vi "DC_Overvoltage_v3.vi"(4 "Polarity":enum16{"Positive", "Negative"}(ring), 5 "Write Task":string="BONTS-93-DC_Link_Input", 6 "# of Channels In":enum16{"1", "2"}(ring), 7 "Read Task":string="BONTS-93-Faults", 8 "error in":errorcluster, 10 "Fault High Threshold":dbl=3.0, 11 "Fault Low Threshold":dbl=0.2) -> (0 "error out":errorcluster, 3 "TS Results":dbl[](array[numeric]))   [LabVIEW 2021]
uses:
  <vilib>/DAQmx/write.llb/DAQmx Write (Analog 1D DBL NChan 1Samp).vi
  <vilib>/DAQmx/read.llb/DAQmx Read (Analog 1D DBL NChan 1Samp).vi
  <vilib>/DAQmx/miscellaneous.llb/DAQmx Fill In Error Info.vi
panel:
  out "Hysteresis":dbl
  out "Fault Out":dbl[](array[numeric]) format="%0.2f"
  in  "Starting Voltage":dbl=4.0
  out "VDC Fault OFF":dbl[](array[numeric])
  in  "Max Voltage":dbl=5.2
  out "VDC Fault ON":dbl[](array[numeric])
  in  "Increments":i32=1000
  # "OV Fault"
  # "Hysteresis"
  # "Fault A"
  # "Fault B"
  # "Fault C"
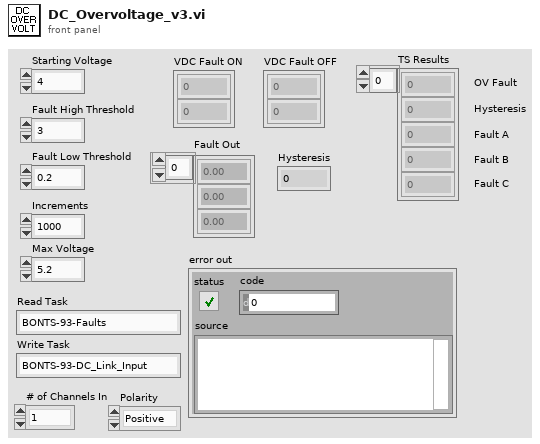
[diagram p1: front panel]
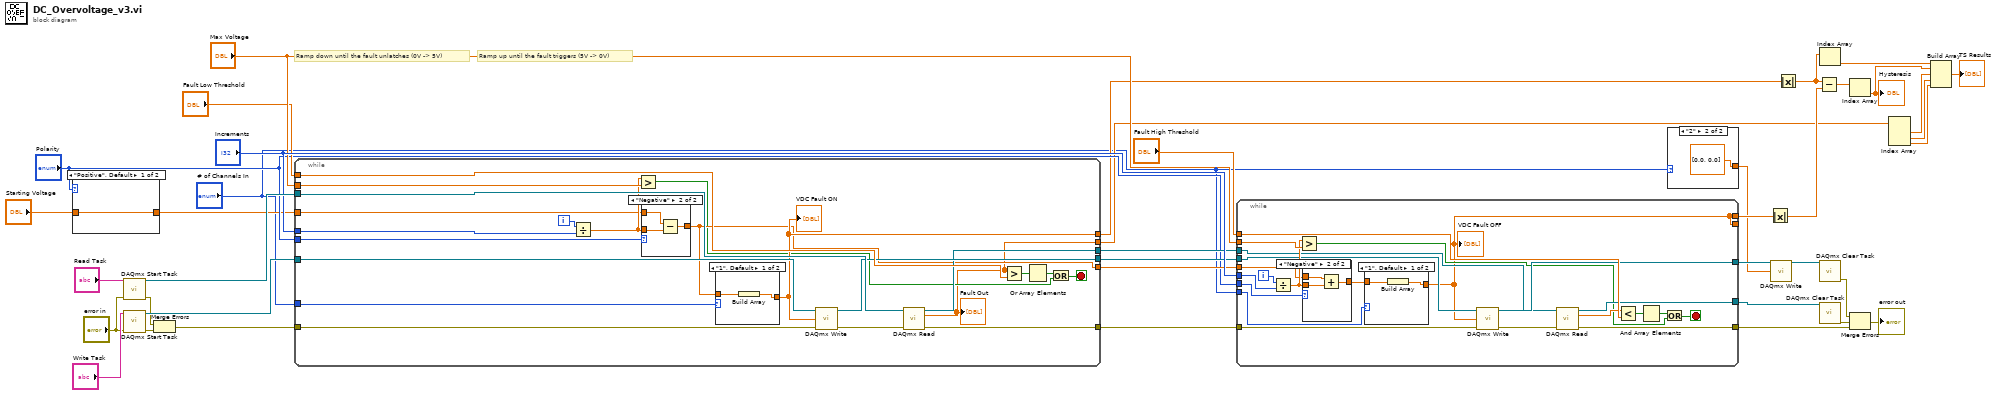
[diagram p0: block diagram]
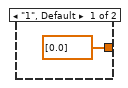
[diagram p2: hidden frame]
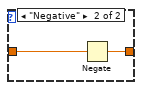
[diagram p3: hidden frame]
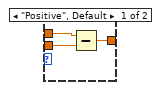
[diagram p4: hidden frame]
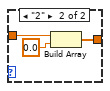
[diagram p5: hidden frame]
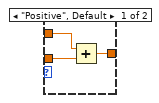
[diagram p6: hidden frame]
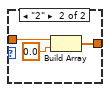
[diagram p7: hidden frame]
diagram:
  # "Ramp down until the fault unlatches (0V -> 5V)"
  # "Ramp up until the fault triggers (5V -> 0V)"
  n1 = case shown="\"Positive\", Default" "Polarity" {
    tunnel: "Starting Voltage" -> [w41 w43]
    tunnel: [w41 w42] -> w15
    frame "Positive", Default {
    }
    frame "Negative" {
      n2 = Negate(x=w43) -> (-x=w42:dbl)
    }
  }
  n3 = call <vilib>:"DAQmx Start Task.vi"("task/channels in"="Read Task", "error in"="error in") -> ("task out"=w37:refnum<k21>, "error out"=w28:errorcluster)  [unwired: 12 in]
  n4 = call <vilib>:"DAQmx Start Task.vi"("task/channels in"="Write Task", "error in"="error in") -> ("task out"=w39:refnum<k21>, "error out"=w27:errorcluster)  [unwired: 12 in]
  n5 = Merge Errors(w28, w27) -> (w29:errorcluster)
  n6 = while {
    tunnel: w37 -> [w65]
    tunnel: w39 -> [w64]
    tunnel: w29 -> [w63]
    tunnel: [w62] -> w25
    tunnel: "Fault Low Threshold" -> [w60]
    tunnel: "Increments" -> [w58]
    tunnel: "Max Voltage" -> [w57]
    tunnel: [w56] -> w24
    tunnel: [w55] -> w23
    tunnel: [w52] -> w22
    tunnel: [w54] -> w13
    tunnel: w15 -> [w51]
    tunnel: "# of Channels In" -> [w50]
    tunnel: "Polarity" -> [w49]
    tunnel: [w44] -> w10
    i -> [w59]
    stop <- w45 stop-if-true
    n7 = Divide(x=w59, y=w58) -> (x/y=w53:dbl)
    n8 = Greater?(x=w53, y=w57) -> (0:w46:bool)
    n9 = case shown="\"Negative\"" w49 {
      tunnel: w53 -> [w67 w71]
      tunnel: [w66 w70] -> w52
      tunnel: w51 -> [w68 w69]
      frame "Positive", Default {
        n10 = Add(x=w68, y=w67) -> (x+y=w66:dbl)
      }
      frame "Negative" {
        n11 = Subtract(x=w69, y=w71) -> (x-y=w70:dbl)
      }
    }
    n12 = case shown="\"1\", Default" w50 {
      tunnel: [w73 w75] -> w54
      tunnel: w52 -> [w72 w74]
      frame "1", Default {
        n13 = Build Array(w72) -> (w73:dbl[])
      }
      frame "2" {
        n14 = Build Array(w74, 0.0 ("element")) -> (w75:dbl[])
      }
    }
    "VDC Fault ON" <- w54
    n15 = call-poly <vilib>:"DAQmx Write.vi"("task/channels in"=w64, "data"=w54, "error in"=w63) -> ("task out"=w56:refnum<k21>, "error out"=w61:errorcluster)  [unwired: 10 in, 1 out]
    n16 = call-poly <vilib>:"DAQmx Read.vi"("task/channels in"=w65, "error in"=w61) -> ("task out"=w55:refnum<k21>, "data"=w44:dbl[], "error out"=w62:errorcluster)  [unwired: 11 in]
    "Fault Out" <- w44
    n17 = Greater?(x=w44, y=w60) -> (0:w48:bool[])
    n18 = Or Array Elements(Boolean array=w48) -> (logical OR=w47:bool)
    n19 = Or(x=w47, y=w46) -> (x .or. y?=w45:bool)
  }
  n20 = while {
    tunnel: [w98] -> w31
    tunnel: "Fault High Threshold" -> [w96]
    tunnel: "Increments" -> [w94]
    tunnel: "Max Voltage" -> [w93]
    tunnel: [w92] -> w34
    tunnel: [w91] -> w21
    tunnel: w25 -> [w90]
    tunnel: w22 -> [w87]
    tunnel: w24 -> [w86]
    tunnel: w23 -> [w85]
    tunnel: [w77] -> _
    tunnel: "# of Channels In" -> [w83]
    tunnel: "Polarity" -> [w82]
    tunnel: [w77] -> w12
    i -> [w95]
    stop <- w78 stop-if-true
    n21 = Divide(x=w95, y=w94) -> (x/y=w88:dbl)
    n22 = Greater?(x=w88, y=w93) -> (0:w79:bool)
    n23 = case shown="\"Negative\"" w82 {
      tunnel: [w101 w102] -> w89
      tunnel: w88 -> [w99 w103]
      tunnel: w87 -> [w100 w104]
      frame "Positive", Default {
        n24 = Subtract(x=w100, y=w99) -> (x-y=w101:dbl)
      }
      frame "Negative" {
        n25 = Add(x=w104, y=w103) -> (x+y=w102:dbl)
      }
    }
    n26 = case shown="\"1\", Default" w83 {
      tunnel: w89 -> [w105 w108]
      tunnel: [w106 w107] -> w77
      frame "1", Default {
        n27 = Build Array(w105) -> (w106:dbl[])
      }
      frame "2" {
        n28 = Build Array(w108, 0.0 ("element")) -> (w107:dbl[])
      }
    }
    "VDC Fault OFF" <- w77
    n29 = call-poly <vilib>:"DAQmx Write.vi"("task/channels in"=w86, "data"=w77, "error in"=w90) -> ("task out"=w91:refnum<k21>, "error out"=w97:errorcluster)  [unwired: 10 in, 1 out]
    n30 = call-poly <vilib>:"DAQmx Read.vi"("task/channels in"=w85, "error in"=w97) -> ("task out"=w92:refnum<k21>, "data"=w84:dbl[], "error out"=w98:errorcluster)  [unwired: 11 in]
    n31 = Less?(x=w84, y=w96) -> (x < y?=w81:bool[])
    n32 = And Array Elements(Boolean array=w81) -> (logical AND=w80:bool)
    n33 = Or(x=w80, y=w79) -> (x .or. y?=w78:bool)
  }
  n34 = case shown="\"2\"" "# of Channels In" {
    tunnel: [dbl[] [0.0] ("data") dbl[] [0.0, 0.0] ("data")] -> w2
    frame "1", Default {
    }
    frame "2" {
    }
  }
  n35 = Absolute Value(x=w12) -> (abs(x)=w14:dbl[])
  n36 = call-poly <vilib>:"DAQmx Write.vi"("task/channels in"=w21, "data"=w2) -> ("task out"=w20:refnum<k21>)  [unwired: 11 in, 2 out]
  n37 = Absolute Value(x=w13) -> (abs(x)=w5:dbl[])
  n38 = Subtract(x=w5, y=w14) -> (x-y=w11:dbl[])
  n39 = Index Array(array=w5) -> (element=w4:dbl)  [unwired: 1 in]
  n40 = call <vilib>:"DAQmx Clear Task.vi"("task in"=w20) -> ("error out"=w33:errorcluster)  [unwired: 14 in]
  n41 = call <vilib>:"DAQmx Clear Task.vi"("task in"=w34) -> ("error out"=w32:errorcluster)  [unwired: 14 in]
  n42 = Index Array(array=w11) -> (element=w6:dbl)  [unwired: 1 in]
  "Hysteresis" <- w6
  n43 = Merge Errors(w33, w32, w31) -> (→"error out":errorcluster)
  n44 = Index Array(array=w10) -> (element #1=w9:dbl, element #2=w8:dbl, element #3=w7:dbl)  [unwired: 3 in]
  n45 = Build Array(w4, w6, w9, w8, w7) -> (→"TS Results":dbl[])
